vi "setSenA.vi"(8 "error in (no error)":errorcluster, 10 "Field Idx":i32[](array[numeric]), 11 "OptStateEsti in":refnum<class "OptStateEsti.lvclass">) -> (0 "error out":errorcluster, 3 "OptStateEsti out":refnum<class "OptStateEsti.lvclass">)   [LabVIEW 2016, in "OptStateEsti.lvclass"]
doc: "Set the sensitivity matrix A based on the array of field index."
uses:
  OptStateEsti.lvclass
  OptStateEsti.lvclass/OptStateEsti.ctl
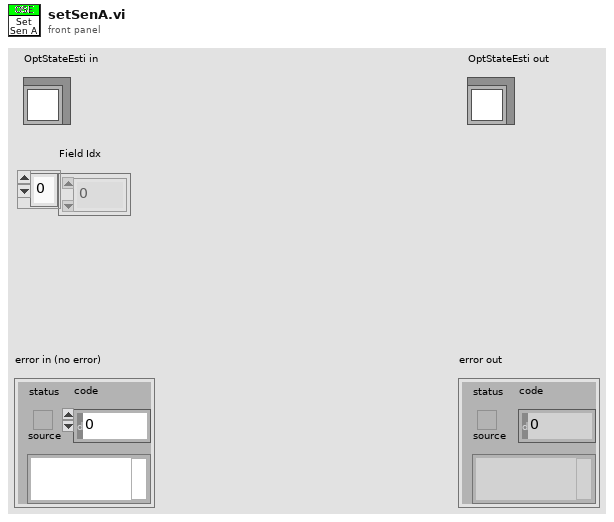
[diagram p1: front panel]
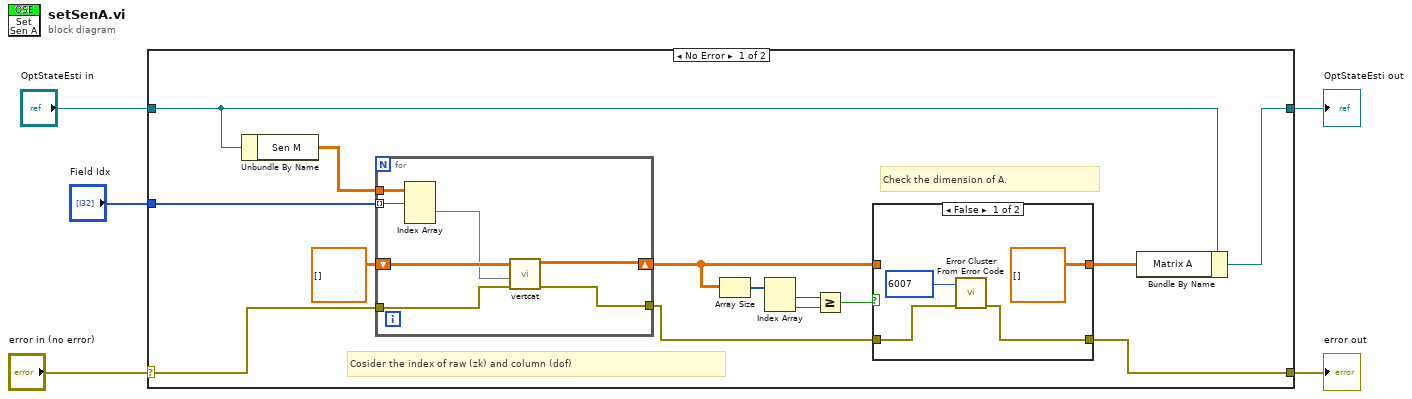
[diagram p0: block diagram]
diagram:
  n1 = case shown="No Error" "error in (no error)" {
    selector: "error in (no error)" -> [w16 w34]
    tunnel: [w9 w34] -> w4
    tunnel: [w6 w33] -> w3
    tunnel: "OptStateEsti in" -> [w7 w33]
    tunnel: "Field Idx" -> [w18 _]
    frame No Error {
      # "Check the dimension of A."
      # "Cosider the index of raw (zk) and column (dof)"
      n2 = Unbundle By Name(w7) -> ("Sen M"=w19:dbl[][][])
      n3 = for {
        tunnel: w19 -> [w32]
        tunnel: w18 -> [w31] mode=indexing
        shift-right: [w29] -> w11
        shift-left: dbl[][] [] ("Stacked 2D Array") -> [w30]
        tunnel: w16 -> [w27]
        tunnel: [w26] -> w10
        n4 = Index Array(array=w32, index (dim 0)=w31) -> (element=w28:dbl[][])  [unwired: 2 in]
        n5 = call "vertcat.vi"("error in (no error)"=w27, "A1"=w28, "A0"=w30) -> ("error out"=w26:errorcluster, "Stacked 2D Array"=w29:dbl[][])  [unwired: 7 in]
      }
      n6 = Array Size(array=w11) -> (size(s)=w15:i32[])
      n7 = Index Array(array=w15) -> (element #1=w14:i32, element #2=w13:i32)  [unwired: 2 in]
      n8 = Greater Or Equal?(x=w14, y=w13) -> (x >= y?=w12:bool)
      n9 = case shown="False" w12 {
        tunnel: [dbl[][] [] ("Stacked 2D Array") w25] -> w8
        tunnel: w11 -> [_ w25]
        tunnel: w10 -> [w21 w24]
        tunnel: [w20 w24] -> w9
        frame False {
          n10 = call <vilib>:"Error Cluster From Error Code.vi"("error in (no error)"=w21, "error code (0)"=6007 ("code")) -> ("error out"=w20:errorcluster)  [unwired: 7 in]
        }
        frame True {
        }
      }
      n11 = Bundle By Name(cluster=w7, "Matrix A"=w8) -> (w6:refnum<class "OptStateEsti.lvclass">)
    }
    frame Error {
    }
  }
  "error out" <- w4
  "OptStateEsti out" <- w3
